vi "ER表头.vi"() -> (3 "ER信息":T1)   [LabVIEW 2017]
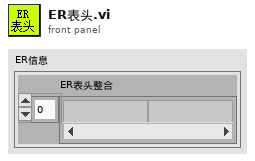
[diagram p1: front panel]
types:
  T1 = typedef "ER信息.ctl" = cluster{"ER表头整合":string[]}
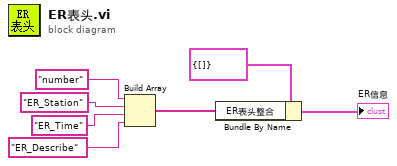
[diagram p0: block diagram]
diagram:
  n1 = Build Array("number", "ER_Station", "ER_Time", "ER_Describe") -> (w1:string[])
  n2 = Bundle By Name(cluster=T1 {"ER表头整合"=[]} ("ER信息"), "ER表头整合"=w1) -> (→"ER信息":T1)
